vi "UnDecorator.vi"(8 "error in (no error)":errorcluster, 11 "DataVer1 in":refnum<class "DataVer1.lvclass">) -> (0 "error out":errorcluster, 2 "DecoratorData Out":refnum<class "Data.lvclass">, 3 "DataVer1 out":refnum<class "DataVer1.lvclass">)   [LabVIEW 2013, in "DataVer1.lvclass"]
uses:
  DataVer1.lvclass
  Data.lvclass/Data.lvclass
  DataVer1.lvclass/DataVer1.ctl
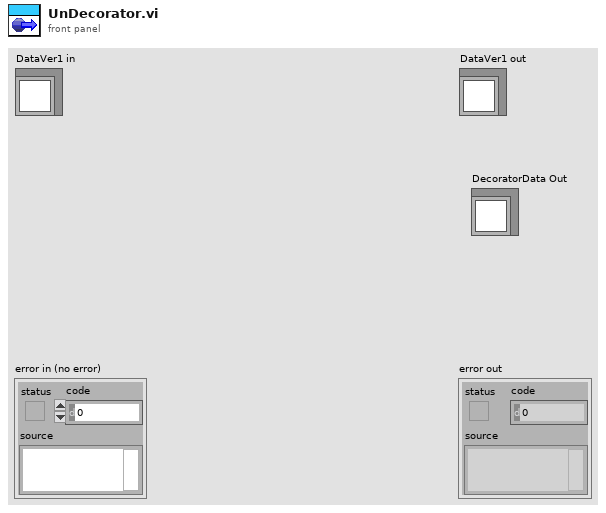
[diagram p1: front panel]
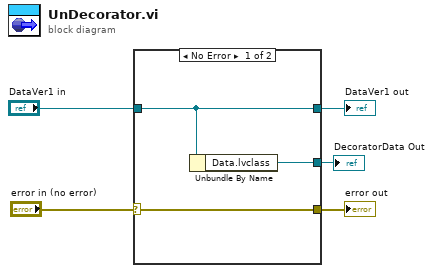
[diagram p0: block diagram]
diagram:
  n1 = case shown="No Error" "error in (no error)" {
    selector: "error in (no error)" -> [w8 w10]
    tunnel: [w8 w10] -> w2
    tunnel: [w7 w9] -> w4
    tunnel: "DataVer1 in" -> [w7 w9]
    tunnel: [w6 _] -> w1
    frame No Error {
      n2 = Unbundle By Name(w7) -> ("Data.lvclass"=w6:refnum<class "Data.lvclass">)
    }
    frame Error {
    }
  }
  "error out" <- w2
  "DataVer1 out" <- w4
  "DecoratorData Out" <- w1
